vi "Total Analysis V.vi"(6 "ROIIndex":i32, 7 "Algorithm":T2, 8 "error in":errorcluster, 9 "ROIList":string[][](array[string]), 10 "AlgParameter":string, 11 "Img in":T1) -> (0 "error out":errorcluster, 1 "DetectResult":variant, 2 "ResultOut":string[][](array[string]), 3 "Img out":T1(plugin-control))   [LabVIEW 2019]
uses:
  Controls/V_Analysis_Type.ctl
  <vilib>/vision/Image Controls.llb/IMAQ Image.ctl
  Controls/Analysis_Setting.ctl
  Ctrl/ROIDataType.ctl
  Controls/Parameter.ctl
  Controls/Color Pattern Match/Analysis Color Pattern Match Parameter.ctl
  Controls/Color Pattern Match/Analysis Color Pattern Match Result.ctl
  Controls/Parttern Match/Analysis_PatternMatch_Parameter.ctl
  Controls/ShapeDectect/Analysis_ShapeDectect_Parameter.ctl
  Controls/ShapeDectect/V_ShapeDectectResult.ctl
  Controls/Geometric Match/Analysis_Geometric PatternMatch_Parameter.ctl
  <vilib>/vision/Pattern Matching.llb/IMAQ Match Range Setting.ctl
  Controls/Geometric Match/Analysis_GeomatricPatternMatch_Result.ctl
  <vilib>/vision/Pattern Matching.llb/IMAQ GM Match Report.ctl
  Controls/Area Check/Area Check_Parameter.ctl
  Controls/Area Check/Area Check_Result.ctl
  c292a3e5-1dec-475a-948c-a0d3e3a21fce.vi
  3bead492-4bfc-46fa-8515-9b4c6ed86bb7.vi
  97097489-2b30-4f47-93f9-e96fbb7cc878.vi
  06c0f7df-6c8d-492f-a42f-5d0db207349b.vi
  5fd81e48-3fa8-4848-b962-4fc8e006ef46.vi
  8e120dce-80e1-4dc2-b1db-1ca67b619174.vi
  24425a9f-bc4e-44c4-80c2-167cb5b99238.vi
  <vilib>/JDP Science/JSONtext/JSON text to Variant.vi
  <vilib>/vision/NI_Vision_Development_Module.lvlib
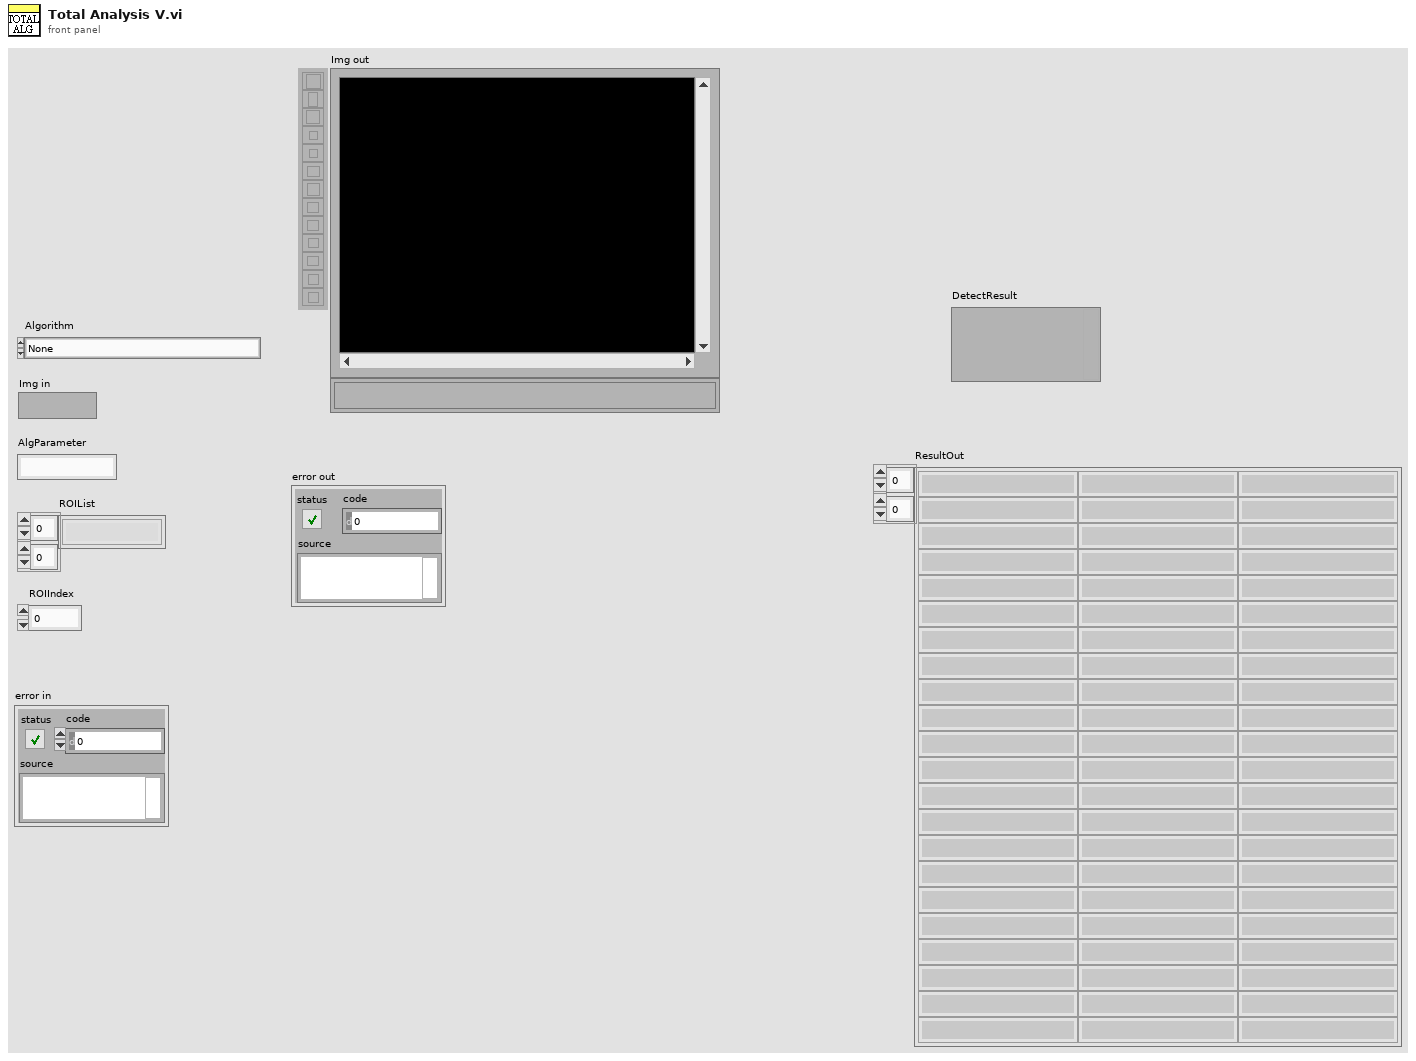
[diagram p1: front panel]
types:
  T1 = typedef "IMAQ Image.ctl" = refnum<image>
  T2 = typedef "V_Analysis_Type.ctl" = enum16{"None", "C_Color Pattern Matching", "G_PatternMatching", "G_ShapeDectect", "G_GeometricMatch", "B_Area Check"}
  T3 = typedef "Parameter.ctl" = enum16{"Initialize", "Write", "Read", "WriteAll", "Save", "Load"}
  T4 = typedef "ROIDataType.ctl" = cluster{"Global Rectangle":i32[], "Contours":cluster{"Contour Type":u32, "ROI Type":u32, "Points":i32[]}[]}
  T5 = typedef "Analysis Color Pattern Match Result.ctl" = cluster{"Number of Matches":i32, "Matches out":cluster{"Position":cluster{"x":sgl, "y":sgl}, "Angle":sgl, "Scale":sgl, "Score":sgl, "Bounding Box":cluster{"x":sgl, "y":sgl}[]}[], "Calibrated Matches":cluster{"Position":cluster{"x":sgl, "y":sgl}, "Angle":sgl, "Scale":sgl, "Score":sgl, "Bounding Box":cluster{"x":sgl, "y":sgl}[]}[], "ROI Descriptor":T6, "ROIName":string}
  T6 = typedef "ROI Descriptor" = cluster{"Global Rectangle":i32[], "Contours":cluster{"ID":enum32{"External", "Internal"}, "Type":u32, "Coordinates":i32[]}[]}
  T7 = typedef "Analysis Color Pattern Match Parameter.ctl" = cluster{"IgnoreBlack And White":enum16{"Disable", "IgnoreBlack", "IgnoreWhite", "IgnoreBlack And White"}, "Match Saturation Threshold":i32, "Minimum Match Score":i32, "Color Score Weight":i32, "Color Sensitivity":u32, "Search Strategy":u32, "Match Offset":cluster{"X":dbl, "Y":dbl}, "Number of Matches to Find":i32, "AngleRange+/-":dbl, "Sub-Pixel Accuracy":bool, "ROI Descriptor":T6, "TemplatePath":string, "Match Mode":enum16{"Shift Invariant", "Rotation Invariant"}}
  T8 = typedef "Analysis_ShapeDectect_Parameter.ctl" = cluster{"Enum_ShapeType":enum16{"Circles", "Ellipses", "Lines", "Rectangles"}, "MaxParticle":i32, "Descriptor":cluster{"Set 1":dbl, "Set 2":dbl, "Set 3":dbl, "Set 4":dbl}, "Match Options":cluster{"Rotation":bool, "Scale":bool, "Occlusion":bool, "Range Settings":cluster{"Match Constraints":u32, "Min":dbl, "Max":dbl}[]}, "Curve Parameters":cluster{"Extraction Mode":u32, "Edge Threshold":i32, "Edge Filter Size":u32, "Min Length":i32, "Row Search Step Size":i32, "Col Search Step Size":i32, "Max Endpoint Gap":i32, "Closed":bool, "Subpixel":bool}, " score":dbl}
  T9 = typedef "Analysis_GeomatricPatternMatch_Result.ctl" = cluster{"Number of Matches":i32, "Matches (pixel)":T10[], "Matches (real-world)":T10[], "Data out":T4, "ROIName":string}
  T10 = typedef "IMAQ GM Match Report.ctl" = cluster{"Position":cluster{"x":sgl, "y":sgl}, "Angle":sgl, "Scale":sgl, "Score":sgl, "Bounding Box":cluster{"x":sgl, "y":sgl}[], "Contrast Reversed":bool, "Occlusion %":sgl, "Template Target Curve Score":sgl, "Target Template Curve Score":sgl, "Correlation Score":sgl}
  T11 = typedef "Analysis_Geometric PatternMatch_Parameter.ctl" = cluster{"Curve Extraction":cluster{"Extraction Mode":u32, "Edge Threshold":i32, "Edge Filter Size":u32, "Min Length":i32, "Row Search Step Size":i32, "Column Search Step Size":i32, "Max Endpoint Gap":i32, "Closed":bool, "Subpixel":bool}, "X Position Offset":i32, "Y Position Offset":i32, "Match Parameters":cluster{"Number of Matches Requested":i32, "Minimum Match Score":sgl, "Angle Ranges":cluster{"Start Angle":sgl, "End Angle":sgl}[]}, "Template path":string, "Range Settings":T12[], "Match Mode":cluster{"Rotation":bool, "Scale":bool, "Occlusion":bool, "Reserved":bool, "Reserved":bool, "Reserved":bool}}
  T12 = typedef "IMAQ Match Range Setting.ctl" = cluster{"Match Constraints":u32, "Min":dbl, "Max":dbl}
  T13 = typedef "Area Check_Result.ctl" = cluster{"AreaDataOut":cluster{"AreaDataOut":cluster{"Rectangle":T14, "Particle Measurements (Pixels)":dbl[][]}}[], "Percent":dbl[], "Item?":bool, "ROI":i32[]}
  T14 = typedef "IMAQ Rectangle" = cluster{"Left":i32, "Top":i32, "Right":i32, "Bottom":i32, "Rotation":dbl}
  T15 = typedef "Area Check_Parameter.ctl" = cluster{"Check Type":enum16{"Black Item White Ground", "White Item Black Ground"}, "NoItem":dbl}
  T16 = typedef "Analysis_Setting.ctl" = cluster{"PreProcess":T2, "Parameter":string}
  T17 = typedef "ParameterData.ctl" = cluster{"Rotate Angle":dbl, "Rotate?":bool, "Calibration File Path":string, "Cal?":bool}
  T18 = typedef "Image Type" = u32
  T19 = cluster{"Position":cluster{"x":sgl, "y":sgl}, "Angle":sgl, "Scale":sgl, "Score":sgl, "Bounding Box":cluster{"x":sgl, "y":sgl}[]}[]
  T20 = typedef "Analysis_PatternMatch_Parameter.ctl" = cluster{"Algorithm":i32, "Match Parameters":cluster{"Number of Matches Requested":i32, "Minimum Match Score":sgl, "Angle Ranges":cluster{"Start Angle":sgl, "End Angle":sgl}[]}, "ROI Descriptor":T6, "Advanced Options":cluster{"Item":u16, "Value":dbl}[], "Template path":string, "XOffset":i32, "YOffset":i32}
  T21 = typedef "Analysis_PatternMatch_Result.ctl" = cluster{"Position":cluster{"x":sgl, "y":sgl}, "Angle":sgl, "Scale":sgl, "Score":sgl, "Bounding Box":cluster{"x":sgl, "y":sgl}[]}
  T22 = typedef "V_ShapeDectectResult.ctl" = cluster{"ResultOut":variant, "DectectItem":i32, "Data out":T4, "ROIName":string}
  T23 = cluster{"AreaDataOut":cluster{"Rectangle":T14, "Particle Measurements (Pixels)":dbl[][]}}[]
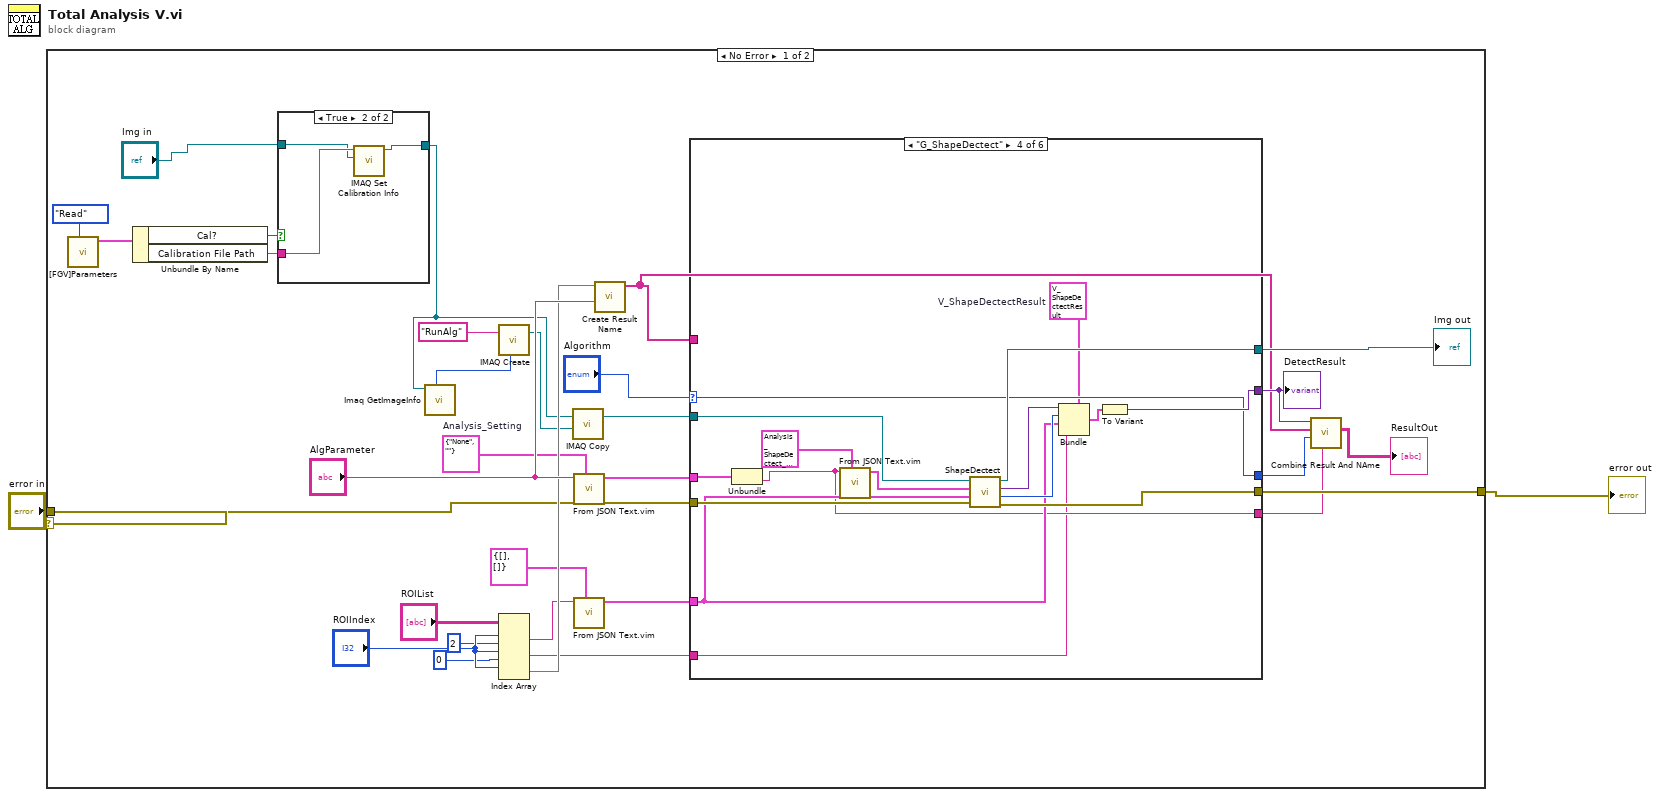
[diagram p0: block diagram]
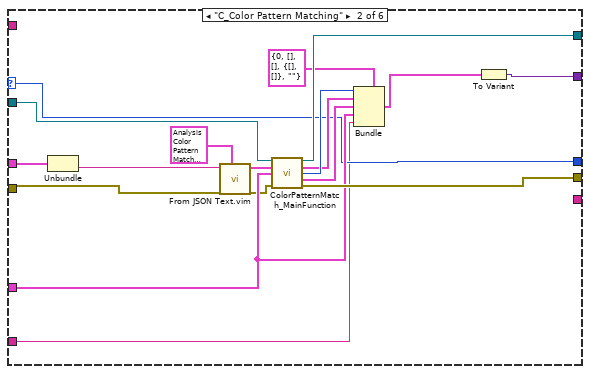
[diagram p4: hidden frame]
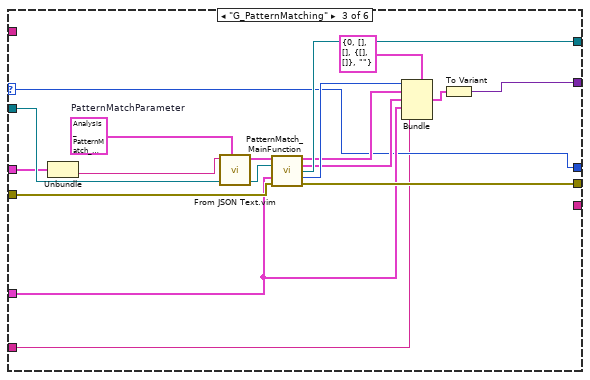
[diagram p5: hidden frame]
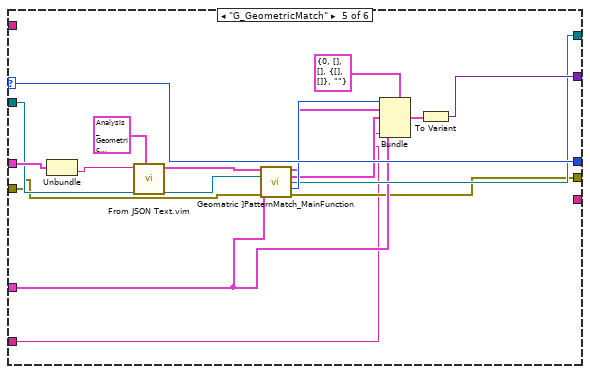
[diagram p6: hidden frame]
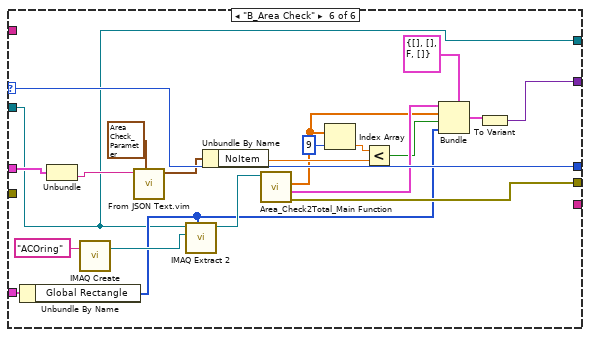
[diagram p7: hidden frame]
diagram:
  n1 = case shown="No Error" "error in" {
    tunnel: [w32 w128] -> w2
    tunnel: "error in" -> [w19 w128]
    frame No Error {
      w20 = T16 {"PreProcess"=enum."None", "Parameter"=""}  # Analysis_Setting
      n2 = call "[FGV]Parameters.vi"("Parameter"=Parameter."Read") -> ("ParameterData Out"=w12:T17)  [unwired: 9 in, 1 out]
      n3 = Unbundle By Name(w12) -> ("Cal?"=w3:bool, "Calibration File Path"=w11:string)
      n4 = case shown="True" w3 {
        tunnel: "Img in" -> [w34 w36]
        tunnel: w11 -> [_ w37]
        tunnel: [w34 w35] -> w9
        frame False {
        }
        frame True {
          n5 = call "IMAQ Set Calibration Info"("Image Dst"=w36, "Image Src"=w37) -> ("Calibrated Image"=w35:T1)  [unwired: 8 in, 1 out]
        }
      }
      n6 = call "Imaq GetImageInfo"("Image"=w9) -> ("Image Type"=w21:T18)  [unwired: 3 in, 7 out]
      n7 = call "IMAQ Create"("Image Name"="RunAlg", "Image Type"=w21) -> ("New Image"=w22:T1)  [unwired: 3 in, 1 out]
      n8 = Index Array(array="ROIList", index (row) #1="ROIIndex", index (col) #1=2 ("disabled index (col)"), index (row) #2="ROIIndex", index (col) #2=0 ("disabled index (col)"), index (row) #3="ROIIndex") -> (element #1=w26:string, element #2=w28:string, element #3=w31:string[])  [unwired: 1 in]
      n9 = call "IMAQ Copy"("Image Dst"=w22, "Image Src"=w9) -> ("Image Dst Out"=w14:T1)  [unwired: 4 in, 1 out]
      n10 = call "From JSON Text.vim"("Data Type and Default Value"=w20, "JSON"="AlgParameter") -> ("Data out"=w29:T16)  [unwired: 8 in, 1 out]
      n11 = call "From JSON Text.vim"("Data Type and Default Value"=T4 {"Global Rectangle"=[], "Contours"=[]} ("ROI DataType"), "JSON"=w26) -> ("Data out"=w15:T4)  [unwired: 8 in, 1 out]
      n12 = call "Create Result Name.vi"("AlgSet"="AlgParameter", "ROIList"=w31) -> ("AlgResultName"=w6:string[])  [unwired: 9 in]
      n13 = case shown="\"G_ShapeDectect\"" "Algorithm" {
        selector: "Algorithm" -> [w39 w42 w59 w76 w102 w124]
        tunnel: w14 -> [_ w56 w73 w81 w101 w107]
        tunnel: w15 -> [_ w43 w62 w78 w93 w119]
        tunnel: [_ w55 w65 w89 w94 w107] -> w17
        tunnel: w28 -> [_ w40 w57 w75 w90 _]
        tunnel: w29 -> [_ w52 w71 w86 w106 w127]
        tunnel: [w38 w46 w68 w82 w92 w122] -> w32
        tunnel: w19 -> [w38 w41 w64 w83 w91 _]
        tunnel: [_ w44 w58 w79 w97 w120] -> w7
        tunnel: w6 -> [_ _ _ _ _ _]
        tunnel: [w39 w42 w59 w76 w102 w124] -> w5
        tunnel: [_ _ _ w77 _ _] -> w4
        frame "None", Default {
        }
        frame "C_Color Pattern Matching" {
          n14 = Unbundle(w52) -> ("Parameter"=w54:string)  [unwired: 1 out]
          n15 = call "From JSON Text.vim"("Data Type and Default Value"=T7 {"IgnoreBlack And White"=enum."IgnoreBlack And White", "Match Saturation Threshold"=80, "Minimum Match Score"=750, "Color Score Weight"=750, "Color Sensitivity"=1, "Search Strategy"=0, "Match Offset"={"X"=0.0, "Y"=0.0}, "Number of Matches to Find"=0, "AngleRange+/-"=0.0, "Sub-Pixel Accuracy"=FALSE, "ROI Descriptor"={"Global Rectangle"=[], "Contours"=[]}, "TemplatePath"="", "Match Mode"=enum."Rotation Invariant"} ("Color Pattern Match"), "JSON"=w54) -> ("Data out"=w51:T7)  [unwired: 8 in, 1 out]
          n16 = call "ColorPatternMatch_MainFunction.vi"("Image in"=w56, "Color Pattern Match"=w51, "ROI Descriptor"=w43, "error in"=w41) -> ("Image Out"=w55:T1, "Matches out"=w48:T19, "Number of Matches"=w49:i32, "Calibrated Matches"=w47:T19, "error out"=w46:errorcluster)  [unwired: 7 in]
          n17 = Bundle(cluster=T5 {"Number of Matches"=0, "Matches out"=[], "Calibrated Matches"=[], "ROI Descriptor"={"Global Rectangle"=[], "Contours"=[]}, "ROIName"=""} ("Color Pattern Matching"), "Number of Matches"=w49, "Matches out"=w48, "Calibrated Matches"=w47, "ROI Descriptor"=w43, "ROIName"=w40) -> (w45:T5)
          n18 = To Variant(anything=w45) -> (Variant=w44:variant)
        }
        frame "G_PatternMatching" {
          w67 = T20 {"Algorithm"=2, "Match Parameters"={"Number of Matches Requested"=1, "Minimum Match Score"=750.0, "Angle Ranges"=[]}, "ROI Descriptor"={"Global Rectangle"=[], "Contours"=[]}, "Advanced Options"=[{"Item"=1, "Value"=1.0}, {"Item"=103, "Value"=1.0}], "Template path"="", "XOffset"=0, "YOffset"=0}  # PatternMatchParameter
          n19 = Unbundle(w71) -> ("Parameter"=w72:string)  [unwired: 1 out]
          n20 = call "From JSON Text.vim"("Data Type and Default Value"=w67, "JSON"=w72) -> ("Data out"=w66:T20)  [unwired: 8 in, 1 out]
          n21 = call "PatternMatch_MainFunction.vi"("PatternMatchParameter"=w66, "Vision_Image In"=w73, "ROI Descriptor"=w62, "error in"=w64) -> ("Matches"=w61:T21[], "Matches (real-world)"=w60:T19, "Image (duplicate)"=w65:T1, "Number of Matches"=w69:i32, "error out"=w68:errorcluster)  [unwired: 7 in]
          n22 = Bundle(cluster=T5 {"Number of Matches"=0, "Matches out"=[], "Calibrated Matches"=[], "ROI Descriptor"={"Global Rectangle"=[], "Contours"=[]}, "ROIName"=""} ("Color Pattern Matching"), "Number of Matches"=w69, "Matches out"=w61, "Calibrated Matches"=w60, "ROI Descriptor"=w62, "ROIName"=w57) -> (w63:T5)
          n23 = To Variant(anything=w63) -> (Variant=w58:variant)
        }
        frame "G_ShapeDectect" {
          w74 = T22 {"ResultOut"=variant, "DectectItem"=0, "Data out"={"Global Rectangle"=[], "Contours"=[]}, "ROIName"=""}  # V_ShapeDectectResult
          n24 = Unbundle(w86) -> ("Parameter"=w77:string)  [unwired: 1 out]
          n25 = call "From JSON Text.vim"("Data Type and Default Value"=T8 {"Enum_ShapeType"=enum."Circles", "MaxParticle"=1, "Descriptor"={"Set 1"=100.0, "Set 2"=10.0, "Set 3"=200.0, "Set 4"=10.0}, "Match Options"={"Rotation"=TRUE, "Scale"=FALSE, "Occlusion"=FALSE, "Range Settings"=[{"Match Constraints"=0, "Min"=0.0, "Max"=360.0}]}, "Curve Parameters"={"Extraction Mode"=0, "Edge Threshold"=75, "Edge Filter Size"=1, "Min Length"=25, "Row Search Step Size"=15, "Col Search Step Size"=15, "Max Endpoint Gap"=10, "Closed"=FALSE, "Subpixel"=FALSE}, " score"=500.0} ("SetParameter"), "JSON"=w77) -> ("Data out"=w84:T8)  [unwired: 8 in, 1 out]
          n26 = call "ShapeDectect.vi"("error in (no error)"=w83, "ROI Descriptor"=w78, "SetParameter"=w84, "Image In"=w81) -> ("error out"=w82:errorcluster, "DectectItem"=w80:i32, "ResultOut"=w88:variant, "Image Out"=w89:T1)  [unwired: 4 in]
          n27 = Bundle(cluster=w74, "ResultOut"=w88, "DectectItem"=w80, "Data out"=w78, "ROIName"=w75) -> (w87:T22)
          n28 = To Variant(anything=w87) -> (Variant=w79:variant)
        }
        frame "G_GeometricMatch" {
          n29 = Unbundle(w106) -> ("Parameter"=w105:string)  [unwired: 1 out]
          n30 = call "From JSON Text.vim"("Data Type and Default Value"=T11 {"Curve Extraction"={"Extraction Mode"=0, "Edge Threshold"=75, "Edge Filter Size"=1, "Min Length"=25, "Row Search Step Size"=15, "Column Search Step Size"=15, "Max Endpoint Gap"=10, "Closed"=FALSE, "Subpixel"=FALSE}, "X Position Offset"=0, "Y Position Offset"=0, "Match Parameters"={"Number of Matches Requested"=1, "Minimum Match Score"=750.0, "Angle Ranges"=[]}, "Template path"="", "Range Settings"=[], "Match Mode"={"Rotation"=TRUE, "Scale"=FALSE, "Occlusion"=FALSE, "Reserved"=FALSE, "Reserved"=FALSE, "Reserved"=FALSE}} ("Cluster"), "JSON"=w105) -> ("Data out"=w103:T11)  [unwired: 8 in, 1 out]
          n31 = call "Geomatric ]PatternMatch_MainFunction.vi"("Geomatric Match Parameter"=w103, "Vision_Image In"=w101, "ROI Descriptor"=w93, "error in"=w91) -> ("Matches (pixel)"=w99:T10[], "Matches (real-world)"=w98:T10[], "Image (duplicate)"=w94:T1, "Number of Matches"=w100:i32, "error out"=w92:errorcluster)  [unwired: 7 in]
          n32 = Bundle(cluster=T9 {"Number of Matches"=0, "Matches (pixel)"=[], "Matches (real-world)"=[], "Data out"={"Global Rectangle"=[], "Contours"=[]}, "ROIName"=""} ("GeomatricMatchResult"), "Number of Matches"=w100, "Matches (pixel)"=w99, "Matches (real-world)"=w98, "Data out"=w93, "ROIName"=w90) -> (w96:T9)
          n33 = To Variant(anything=w96) -> (Variant=w97:variant)
        }
        frame "B_Area Check" {
          n34 = Unbundle By Name(w119) -> ("Global Rectangle"=w109:i32[])
          n35 = Unbundle(w127) -> ("Parameter"=w126:string)  [unwired: 1 out]
          n36 = call "IMAQ Create"("Image Name"="ACOring") -> ("New Image"=w118:T1)  [unwired: 4 in, 1 out]
          n37 = call "From JSON Text.vim"("Data Type and Default Value"=T15 {"Check Type"=enum."Black Item White Ground", "NoItem"=0.0} ("cluster"), "JSON"=w126) -> ("Data out"=w116:T15)  [unwired: 8 in, 1 out]
          n38 = call "IMAQ Extract 2"("Optional Rectangle"=w109, "Image Dst"=w118, "Image Src"=w107) -> ("Image Dst Out"=w121:T1)  [unwired: 7 in, 1 out]
          n39 = Unbundle By Name(w116) -> ("NoItem"=w113:dbl)
          n40 = call "Area_Check2Total_Main Function.vi"("img in"=w121) -> ("error out"=w122:errorcluster, "AreaDataOut"=w112:T23, "Array"=w111:dbl[])  [unwired: 7 in, 1 out]
          n41 = Index Array(array=w111, index=9) -> (element=w114:dbl)
          n42 = Less?(x=w114, y=w113) -> (x < y?=w110:bool)
          n43 = Bundle(cluster=T13 {"AreaDataOut"=[], "Percent"=[], "Item?"=FALSE, "ROI"=[]}, "AreaDataOut"=w112, "Percent"=w111, "Item?"=w110, "ROI"=w109) -> (w123:T13)
          n44 = To Variant(anything=w123) -> (Variant=w120:variant)
        }
      }
      "Img out" <- w17
      "DetectResult" <- w7
      n45 = call "Combine Result And NAme.vi"("SetParameter"=w4, "Analysis"=w5, "AlgResultName"=w6, "DataIn"=w7) -> ("ResultOut"=→"ResultOut":string[][])  [unwired: 7 in]
    }
    frame Error {
    }
  }
  "error out" <- w2
